vi "FCI_EON_Outer_Width.vi"(0 "Image":T8(plugin-control), 1 "Reference Edge ROI":T13 {"Contours"."Type" items=["No Selection", "Point", "Line", "Rectangle", "Oval", "Polygon", "Freehand Region", "Annulus", "Unused2", "Unused3", "Broken Line", "Freehand Line", "Rotated Rectangle"]}, 2 "Calibrated Image":T8, 3 "Measurement ROI":T13 {"Contours"."Type" items=["No Selection", "Point", "Line", "Rectangle", "Oval", "Polygon", "Freehand Region", "Annulus", "Unused2", "Unused3", "Broken Line", "Freehand Line", "Rotated Rectangle"]}, 4 "Blob Center":cluster{"Center X":dbl, "Center Y":dbl}, 5 "error in (no error) 2":errorcluster, 6 "Edge Options ROI Ref":T9={"Edge Polarity"=0, "Kernel Size"=3, "Width"=3, "Minimum Edge Strength"=50.0, "Interpolation Type"=enum."Bilinear Fixed", "Data Processing Method"=enum."Average"} {"Edge Polarity" items=["All Edges", "Rising Edges", "Falling Edges"]; "Minimum Edge Strength" format="%.2f"; "Width" step=2; "Kernel Size" step=2}, 7 "Line Options ROI Ref":T11={"Number of Lines"=1, "Type"=enum."First Edge Rake", "Min. Score"=10.0, "Max. Score"=1000.0, "Orientation"=0.0, "Angle Range"=45.0, "Angle Tolerance"=1.0, "Step Size"=3, "Min. SNR (db)"=0.0, "Min. Points (%)"=25.0, "Hough Iterations"=5} {"Min. Points (%)" min=0.0 max=100.0; "Min. SNR (db)" min=0.0; "Max. Score" min=0.0 max=1024.0; "Min. Score" min=0.0 max=1024.0 step=1.0}, 8 "Search Direction ROI 1":u16(ring) items=["Left To Right", "Right To Left", "Top To Bottom", "Bottom To Top"], 10 "Search Direction Ref ROI":u32, 11 "Edge Options ROI 1":T9={"Edge Polarity"=0, "Kernel Size"=3, "Width"=3, "Minimum Edge Strength"=50.0, "Interpolation Type"=enum."Zero Order", "Data Processing Method"=enum."Average"} {"Edge Polarity" items=["All Edges", "Rising Edges", "Falling Edges"]; "Minimum Edge Strength" format="%.2f"; "Width" step=2; "Kernel Size" step=2}) -> (14 "EON Outer width Real World":sgl, 15 "Overlay Line Arrows":T1, 19 "error IO":errorcluster)   [LabVIEW 2019, in "Algorithm.lvclass"]
uses:
  FrameworkOverrides/Algorithm.lvclass
  <vilib>/vision/NI_Vision_Development_Module.lvlib
  <vilib>/vision/Measure.llb/Edge Polarity.ctl
  <vilib>/vision/Measure.llb/Edge Options.ctl
  <vilib>/vision/Measure.llb/Straight Edge Process.ctl
  <vilib>/vision/Measure.llb/Straight Edge Options.ctl
  <vilib>/vision/Image Controls.llb/IMAQ Image.ctl
  <vilib>/vision/Measure.llb/Edge New.ctl
  <vilib>/vision/Measure.llb/Search Line.ctl
panel:
  out "Second Overlay Line":T2
  out "First Overlay Line":T3
  out "Search Lines":T4[](array[typedef]) {"Edge Info"."Distance (Real-World)" format="%.2f"; "Edge Info"."Location (Real-World)"."Y" format="%.2g"; "Edge Info"."Location (Real-World)"."X" format="%.2f"; "Edge Info"."Noise" format="%.2f"; "Edge Info"."Location (Pixel)"."Y" format="%.2g"; "Edge Info"."Location (Pixel)"."X" format="%.2f"; "Edge Info"."Strength" format="%.2f"; "Edge Info"."Distance (Pixel)" format="%.2f"}
  out "Perpendicular Lines":T6(array[cluster])=[{{"X"=55.0, "Y"=48.0}, {"X"=263.0, "Y"=104.0}}, {{"X"=53.0, "Y"=53.0}, {"X"=262.0, "Y"=109.0}}, {{"X"=52.0, "Y"=58.0}, {"X"=261.0, "Y"=113.0}}, {{"X"=51.0, "Y"=62.0}, {"X"=259.0, "Y"=118.0}}, {{"X"=49.0, "Y"=67.0}, {"X"=258.0, "Y"=123.0}}, {{"X"=48.0, "Y"=72.0}, {"X"=257.0, "Y"=128.0}}, {{"X"=47.0, "Y"=77.0}, {"X"=255.0, "Y"=133.0}}, {{"X"=46.0, "Y"=82.0}, {"X"=254.0, "Y"=138.0}}, {{"X"=44.0, "Y"=87.0}, {"X"=253.0, "Y"=142.0}}, {{"X"=43.0, "Y"=91.0}, {"X"=252.0, "Y"=147.0}}, {{"X"=42.0, "Y"=96.0}, {"X"=250.0, "Y"=152.0}}] {"?"."Y" format="%.2f"; "?"."X" format="%.2f"; "?"."Y" format="%.2f"; "?"."X" format="%.2f"}
  out "output cluster":T7
  out "Angle (Pixel)":dbl
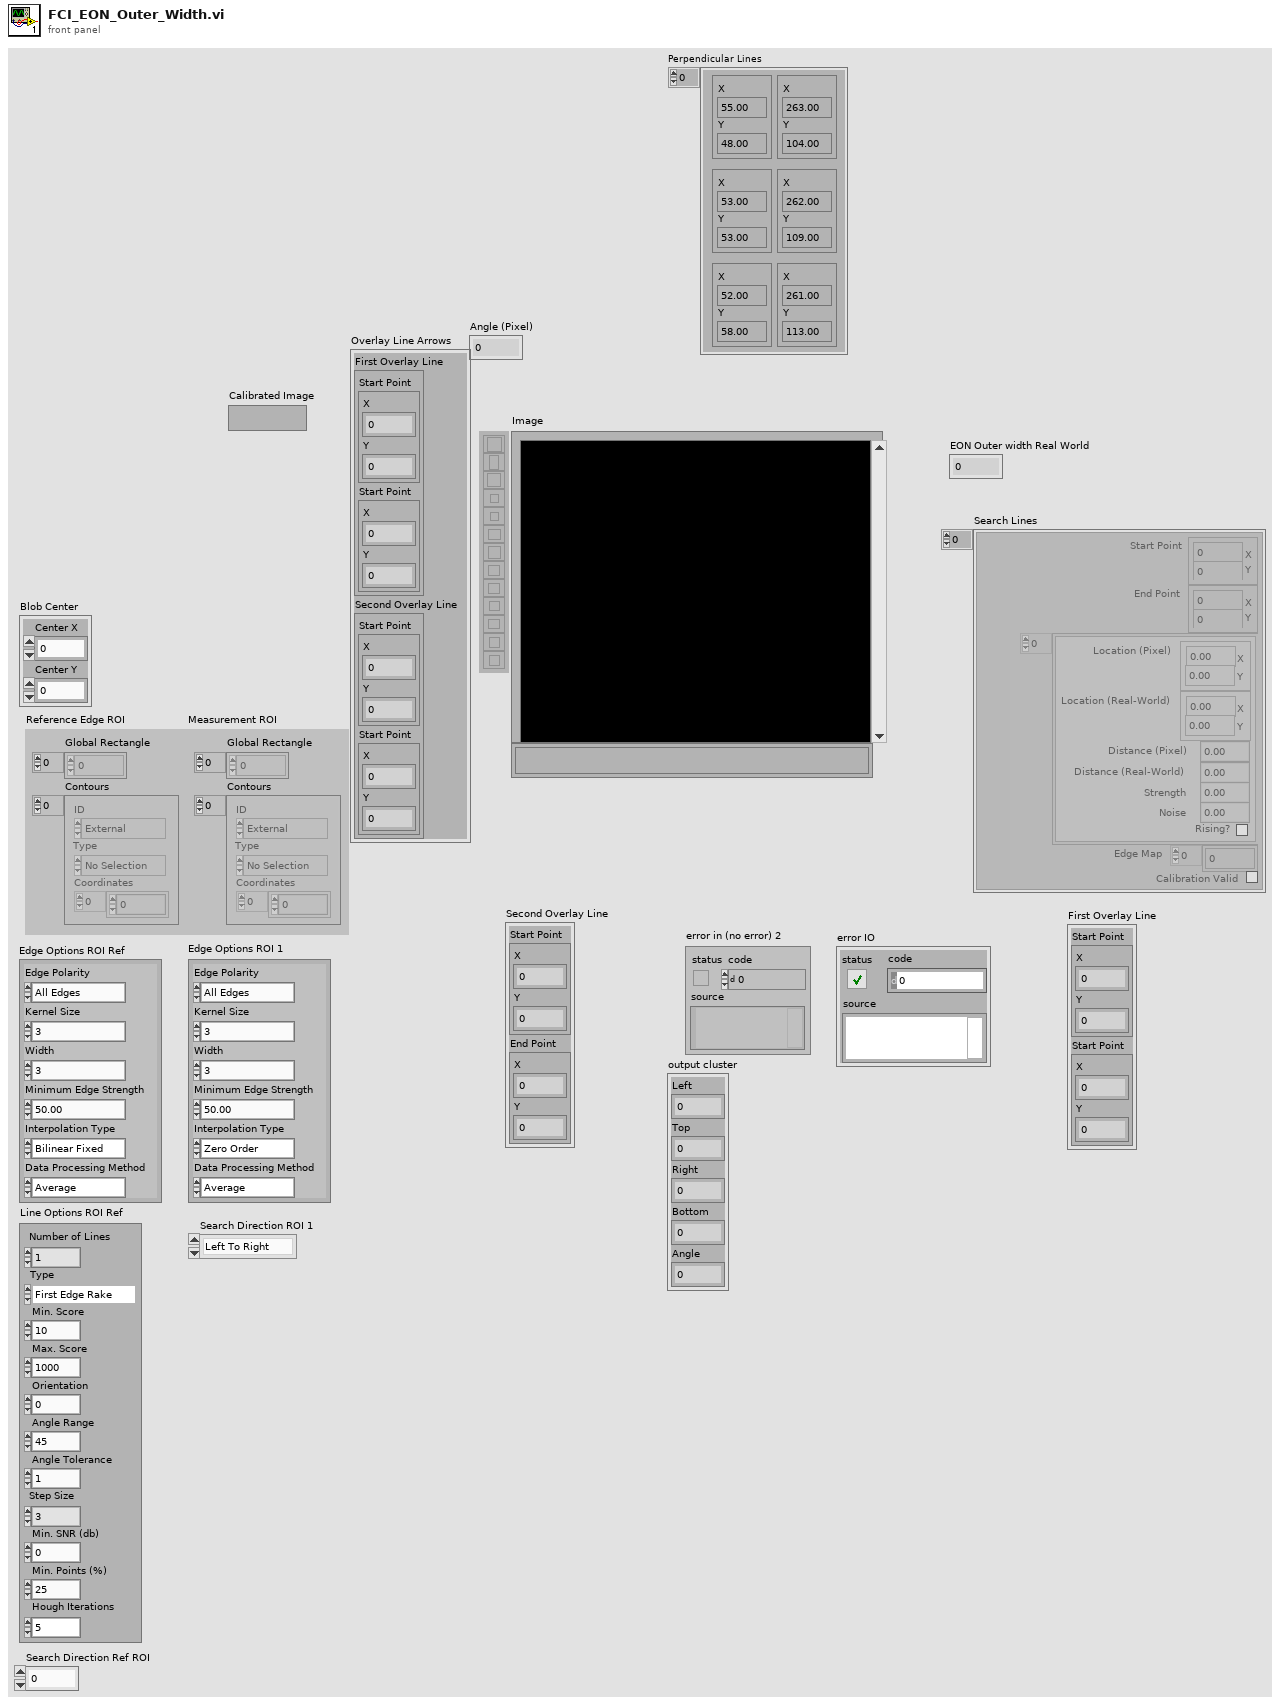
[diagram p1: front panel]
types:
  T1 = cluster{"First Overlay Line ":cluster{"Start Point":cluster{"X":sgl, "Y":sgl}, "Start Point":cluster{"X":sgl, "Y":sgl}}, "Second Overlay Line ":cluster{"Start Point":cluster{"X":sgl, "Y":sgl}, "Start Point":cluster{"X":sgl, "Y":sgl}}}
  T2 = cluster{"Start Point":cluster{"X":sgl, "Y":sgl}, "End Point":cluster{"X":sgl, "Y":sgl}}
  T3 = cluster{"Start Point":cluster{"X":sgl, "Y":sgl}, "Start Point":cluster{"X":sgl, "Y":sgl}}
  T4 = typedef "Search Line.ctl" = cluster{"Start Point":cluster{"X":sgl, "Y":sgl}, "End Point":cluster{"X":sgl, "Y":sgl}, "Edge Info":T5[], "Edge Map":dbl[], "Calibration Valid":bool}
  T5 = typedef "Edge New.ctl" = cluster{"Location (Pixel)":cluster{"X":sgl, "Y":sgl}, "Location (Real-World)":cluster{"X":sgl, "Y":sgl}, "Distance (Pixel)":dbl, "Distance (Real-World)":dbl, "Strength":dbl, "Noise":dbl, "Rising?":bool}
  T6 = cluster{cluster{"X":sgl, "Y":sgl}, cluster{"X":sgl, "Y":sgl}}[]
  T7 = cluster{"Left":dbl, "Top":dbl, "Right":dbl, "Bottom":dbl, "Angle":dbl}
  T8 = typedef "IMAQ Image.ctl" = refnum<image>
  T9 = typedef "Edge Options.ctl" = cluster{"Edge Polarity":T10, "Kernel Size":u32, "Width":u32, "Minimum Edge Strength":sgl, "Interpolation Type":enum32{"Zero Order", "Bilinear", "Quadratic", "Cubic", "Bilinear Fixed"}, "Data Processing Method":enum32{"Average", "Median"}}
  T10 = typedef "Edge Polarity.ctl" = u32
  T11 = typedef "Straight Edge Options.ctl" = cluster{"Number of Lines":i32, "Type":T12, "Min. Score":dbl, "Max. Score":dbl, "Orientation":dbl, "Angle Range":dbl, "Angle Tolerance":dbl, "Step Size":u32, "Min. SNR (db)":dbl, "Min. Points (%)":dbl, "Hough Iterations":i32}
  T12 = typedef "Straight Edge Process.ctl" = enum32{"First Edge Rake", "Best Edge Rake", "Hough Edge Rake", "First Edge Projection", "Best Edge Projection"}
  T13 = typedef "ROI Descriptor" = cluster{"Global Rectangle":i32[], "Contours":cluster{"ID":enum32{"External", "Internal"}, "Type":u32, "Coordinates":i32[]}[]}
  T14 = cluster{"Search Direction":u32, "Edge Options":T9, "Show Search Area":bool, "Show Search Lines":bool, "Show Edges Found":bool, "Show Result":bool, "Search Area Color":u32, "Search Lines Color":u32, "Edge Locations Color":u32, "Result Color":u32, "Overlay Group Name":string}
  T15 = typedef "IMAQ Rectangle" = cluster{"Left":i32, "Top":i32, "Right":i32, "Bottom":i32, "Rotation":dbl}
  T16 = cluster{"Point1 (Pixels)":cluster{"X":sgl, "Y":sgl}, "Point2 (Pixels)":cluster{"X":sgl, "Y":sgl}, "Point1 (Real-World)":cluster{"X":sgl, "Y":sgl}, "Point2 (Real-World)":cluster{"X":sgl, "Y":sgl}, "Angle (Pixel)":dbl, "Angle (Real-World)":dbl, "Score":dbl, "Straightness":dbl, "Average SNR (db)":dbl, "Calibration Valid":bool}[]
  T17 = cluster{"Point1 (Pixels)":cluster{"X":sgl, "Y":sgl}, "Point2 (Pixels)":cluster{"X":sgl, "Y":sgl}, "Point1 (Real-World)":cluster{"X":sgl, "Y":sgl}, "Point2 (Real-World)":cluster{"X":sgl, "Y":sgl}, "Angle (Pixel)":dbl, "Angle (Real-World)":dbl, "Score":dbl, "Straightness":dbl, "Average SNR (db)":dbl, "Calibration Valid":bool}
  T18 = cluster{"Start Point":cluster{"X":sgl, "Y":sgl}, cluster{"X":sgl, "Y":sgl}}
  T19 = cluster{cluster{"X":sgl, "Y":sgl}, "End Point":cluster{"X":sgl, "Y":sgl}}
  T20 = cluster{"Start Point":cluster{"X":sgl, "Y":sgl}, cluster{"X":sgl, "Y":sgl}, cluster{"X":sgl, "Y":sgl}, "End Point":cluster{"X":sgl, "Y":sgl}}
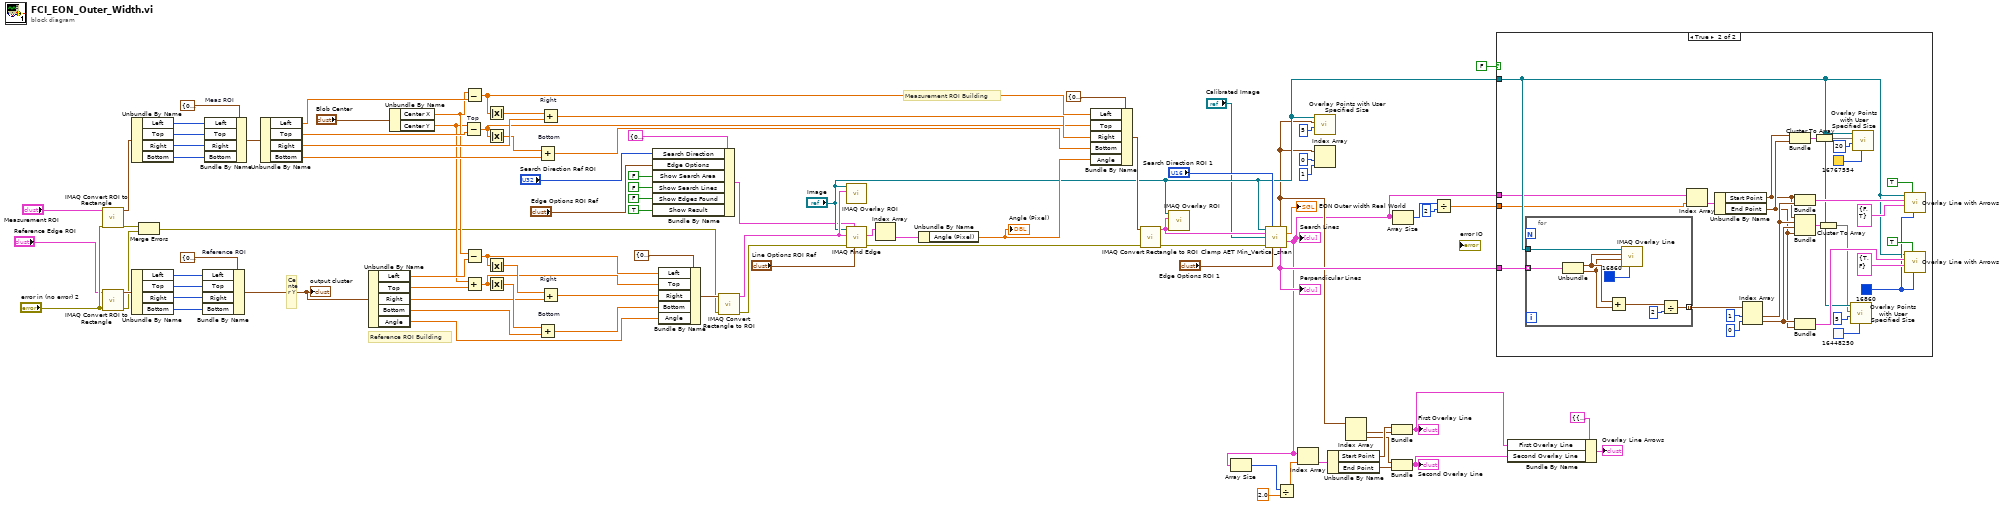
[diagram p0: block diagram]
diagram:
  # "Measurement ROI Building"
  # "Reference ROI Building"
  # "Center Y"
  n1 = call "IMAQ Convert ROI to Rectangle"("error in (no error)"="error in (no error) 2", "ROI Descriptor"="Measurement ROI") -> ("error out"=w38:errorcluster, "Rectangle"=w48:T15)  [unwired: 7 in]
  n2 = call "IMAQ Convert ROI to Rectangle"("error in (no error)"="error in (no error) 2", "ROI Descriptor"="Reference Edge ROI") -> ("error out"=w37:errorcluster, "Rectangle"=w47:T15)  [unwired: 7 in]
  n3 = Unbundle By Name(w48) -> ("Left"=w42:i32, "Top"=w41:i32, "Right"=w40:i32, "Bottom"=w39:i32)
  n4 = Unbundle By Name(w47) -> ("Left"=w46:i32, "Top"=w45:i32, "Right"=w44:i32, "Bottom"=w43:i32)
  n5 = Merge Errors(w38, w37) -> (w36:errorcluster)
  n6 = Bundle By Name "Reference ROI"(cluster=T7 {"Left"=0.0, "Top"=0.0, "Right"=0.0, "Bottom"=0.0, "Angle"=0.0} ("input cluster"), "Left"=w46, "Top"=w45, "Right"=w44, "Bottom"=w43) -> (w62:T7)
  "output cluster" <- w62
  n7 = Bundle By Name "Meas ROI"(cluster=T7 {"Left"=0.0, "Top"=0.0, "Right"=0.0, "Bottom"=0.0, "Angle"=0.0} ("input cluster"), "Left"=w42, "Top"=w41, "Right"=w40, "Bottom"=w39) -> (w60:T7)
  n8 = Unbundle By Name(w60) -> ("Left"=w79:dbl, "Top"=w78:dbl, "Right"=w77:dbl, "Bottom"=w76:dbl)
  n9 = Unbundle By Name(w62) -> ("Left"=w75:dbl, "Top"=w74:dbl, "Right"=w73:dbl, "Bottom"=w72:dbl, "Angle"=w71:dbl)
  n10 = Unbundle By Name("Blob Center") -> ("Center X"=w52:dbl, "Center Y"=w51:dbl)
  n11 = Subtract "Top"(x=w51, y=w78) -> (x-y=w64:dbl)
  n12 = Subtract(x=w52, y=w79) -> (x-y=w89:dbl)
  n13 = Subtract(x=w52, y=w75) -> (x-y=w83:dbl)
  n14 = Add(x=w51, y=w74) -> (x+y=w82:dbl)
  n15 = Absolute Value(x=w89) -> (abs(x)=w91:dbl)
  n16 = Absolute Value(x=w64) -> (abs(x)=w65:dbl)
  n17 = Absolute Value(x=w83) -> (abs(x)=w86:dbl)
  n18 = Absolute Value(x=w82) -> (abs(x)=w85:dbl)
  n19 = Add "Bottom"(x=w65, y=w76) -> (x+y=w87:dbl)
  n20 = Add "Bottom"(x=w85, y=w72) -> (x+y=w80:dbl)
  n21 = Add "Right"(x=w91, y=w77) -> (x+y=w88:dbl)
  n22 = Add "Right"(x=w86, y=w73) -> (x+y=w81:dbl)
  n23 = Bundle By Name(cluster=T14 {"Search Direction"=0, "Edge Options"={"Edge Polarity"=0, "Kernel Size"=3, "Width"=3, "Minimum Edge Strength"=50.0, "Interpolation Type"=enum."Zero Order", "Data Processing Method"=enum."Average"}, "Show Search Area"=FALSE, "Show Search Lines"=FALSE, "Show Edges Found"=FALSE, "Show Result"=TRUE, "Search Area Color"=65280, "Search Lines Color"=255, "Edge Locations Color"=16776960, "Result Color"=16711680, "Overlay Group Name"=""} ("Options"), "Search Direction"="Search Direction Ref ROI", "Edge Options"="Edge Options ROI Ref", "Show Search Area"=FALSE, "Show Search Lines"=FALSE, "Show Edges Found"=FALSE, "Show Result"=TRUE) -> (w18:T14)
  n24 = Bundle By Name(cluster=T7 {"Left"=0.0, "Top"=0.0, "Right"=0.0, "Bottom"=0.0, "Angle"=0.0} ("input cluster"), "Left"=w83, "Top"=w82, "Right"=w81, "Bottom"=w80, "Angle"=w71) -> (w66:T7)
  n25 = call "IMAQ Convert Rectangle to ROI"("error in (no error)"=w36, "Rectangle"=w66) -> ("error out"=w70:errorcluster, "ROI Descriptor"=w59:T13)  [unwired: 7 in]
  n26 = call "IMAQ Overlay ROI"("ROI Descriptor"=w59, "Image"="Image") -> ()  [unwired: 8 in, 2 out]
  n27 = call "IMAQ Find Edge"("Line Fit Options"="Line Options ROI Ref", "Options"=w18, "error in (no error)"=w70, "ROI Descriptor"=w59, "Image"="Image") -> ("error out"=w57:errorcluster, "Straight Edges"=w68:T16)  [unwired: 3 in, 2 out]
  n28 = Index Array(array=w68) -> (element=w67:T17)  [unwired: 1 in]
  n29 = Unbundle By Name(w67) -> ("Angle (Pixel)"=w26:dbl)
  "Angle (Pixel)" <- w26
  n30 = Bundle By Name(cluster=T7 {"Left"=0.0, "Top"=0.0, "Right"=0.0, "Bottom"=0.0, "Angle"=0.0} ("input cluster"), "Left"=w89, "Top"=w64, "Right"=w88, "Bottom"=w87, "Angle"=w26) -> (w24:T7)
  n31 = call "IMAQ Convert Rectangle to ROI"("error in (no error)"=w57, "Rectangle"=w24) -> ("error out"=w56:errorcluster, "ROI Descriptor"=w54:T13)  [unwired: 7 in]
  n32 = call "IMAQ Overlay ROI"("ROI Descriptor"=w54, "Image"="Image") -> ()  [unwired: 8 in, 2 out]
  n33 = call "Clamp AET Min_Vertical_shan.vi"("Image"="Image", "Scanning axis"="Search Direction ROI 1", "ROI Descriptor"=w54, "Calibrated Image"="Calibrated Image", "error in (no error)"=w56, "Edge Options"="Edge Options ROI 1") -> ("Edge Coordinates"=w3:cluster{"X":sgl, "Y":sgl}[], "Distance"=→"EON Outer width Real World":sgl, "Search Lines"=w2:T4[], "Perpendicular Lines"=w25:T6)  [unwired: 3 in, 3 out]
  "Perpendicular Lines" <- w25
  "Search Lines" <- w2
  n34 = Array Size(array=w2) -> (size(s)=w5:i32)
  n35 = Divide(x=w5, y=2.0) -> (x/y=w4:dbl)
  n36 = Index Array(array=w2, index=w4) -> (element=w14:T4)
  n37 = call "Overlay Points with User Specified Size.vi"("Point Diameter (5)"=u32 5, "Points"=w3, "Image In"="Image") -> ()  [unwired: 7 in, 2 out]
  n38 = Index Array(array=w3, index #1=0 ("index"), index #2=1 ("index")) -> ()  [unwired: 2 out]
  n39 = Unbundle By Name(w14) -> ("Start Point"=w13:cluster{"X":sgl, "Y":sgl}, "End Point"=w10:cluster{"X":sgl, "Y":sgl})
  n40 = Index Array(array=w3) -> (element #1=w12:cluster{"X":sgl, "Y":sgl}, element #2=w11:cluster{"X":sgl, "Y":sgl})  [unwired: 2 in]
  n41 = Bundle("Start Point"=w13, w12) -> (w8:T18)  [unwired: 1 in]
  "First Overlay Line" <- w8
  n42 = Bundle(w11, "End Point"=w10) -> (w7:T19)  [unwired: 1 in]
  "Second Overlay Line" <- w7
  n43 = Array Size(array=w2) -> (size(s)=w22:i32)
  n44 = Divide(x=w22, y=2) -> (x/y=w20:dbl)
  n45 = case shown="True" FALSE {
    tunnel: w25 -> [_ w109]
    tunnel: "Image" -> [_ w102]
    tunnel: w2 -> [_ w100]
    tunnel: w20 -> [_ w97]
    frame False {
    }
    frame True {
      w110 = u32 16860 ("Color")
      n46 = for {
        tunnel: w109 -> [w126] mode=indexing
        tunnel: w102 -> [w125]
        tunnel: [w120] -> w108 mode=indexing
        n47 = Unbundle(w126) -> (w124:cluster{"X":sgl, "Y":sgl}, w123:cluster{"X":sgl, "Y":sgl})
        n48 = Add(x=w124, y=w123) -> (x+y=w122:cluster{"X":sgl, "Y":sgl})
        n49 = call "IMAQ Overlay Line"("Color"=u32 16860, "End Point"=w123, "Start Point"=w124, "Image"=w125) -> ()  [unwired: 6 in, 2 out]
        n50 = Divide(x=w122, y=2) -> (x/y=w120:cluster{"X":sgl, "Y":sgl})
      }
      n51 = Index Array(array=w100, index=w97) -> (element=w99:T4)
      n52 = Unbundle By Name(w99) -> ("Start Point"=w95:cluster{"X":sgl, "Y":sgl}, "End Point"=w96:cluster{"X":sgl, "Y":sgl})
      n53 = Index Array(array=w108, index #1=1 ("index"), index #2=0 ("index")) -> (element #1=w107:cluster{"X":sgl, "Y":sgl}, element #2=w106:cluster{"X":sgl, "Y":sgl})
      n54 = Bundle("Start Point"=w95, "End Point"=w96) -> (w98:T2)  [unwired: 1 in]
      n55 = Bundle("Start Point"=w95, w107) -> (w116:T18)  [unwired: 1 in]
      n56 = Bundle("Start Point"=w95, w107, w106, "End Point"=w96) -> (w118:T20)  [unwired: 1 in]
      n57 = Bundle(w106, "End Point"=w96) -> (w111:T19)  [unwired: 1 in]
      n58 = Cluster To Array(cluster=w98) -> (array=w93:cluster{"X":sgl, "Y":sgl}[])
      n59 = Cluster To Array(cluster=w118) -> (array=w94:cluster{"X":sgl, "Y":sgl}[])
      n60 = call "Overlay Points with User Specified Size.vi"("Color"=u32 16448250, "Point Diameter (5)"=u32 5, "Points"=w94, "Image In"=w102) -> ()  [unwired: 6 in, 2 out]
      n61 = call "Overlay Points with User Specified Size.vi"("Color"=u32 16767554, "Point Diameter (5)"=u32 20, "Points"=w93, "Image In"=w102) -> ()  [unwired: 6 in, 2 out]
      n62 = call <vilib>:"Overlay Line with Arrows.vi"("Color"=w110, "Draw line?"=TRUE, "Arrows"=cluster{"Start point":bool, "End point":bool} {"Start point"=FALSE, "End point"=TRUE}, "Line Coordinates"=w116, "Image In"=w102) -> ()  [unwired: 5 in, 2 out]
      n63 = call <vilib>:"Overlay Line with Arrows.vi"("Color"=w110, "Draw line?"=TRUE, "Arrows"=cluster{"Start point":bool, "End point":bool} {"Start point"=TRUE, "End point"=FALSE}, "Line Coordinates"=w111, "Image In"=w102) -> ()  [unwired: 5 in, 2 out]
    }
  }
  n64 = Bundle By Name(cluster=T1 {"First Overlay Line "={"Start Point"={"X"=0.0, "Y"=0.0}, "Start Point"={"X"=0.0, "Y"=0.0}}, "Second Overlay Line "={"Start Point"={"X"=0.0, "Y"=0.0}, "Start Point"={"X"=0.0, "Y"=0.0}}}, "First Overlay Line"=w8, "Second Overlay Line"=w7) -> (→"Overlay Line Arrows":T1)
